vi "Write ModuleWidth.vi"(8 "error in (no error)":errorcluster, 10 "ModuleWidth":u8, 11 "Linear Barcode in":refnum<class "Linear Barcode.lvclass">) -> (0 "error out":errorcluster, 3 "Linear Barcode out":refnum<class "Linear Barcode.lvclass">)   [LabVIEW 2013, in "BarCodes.lvlib" / "Linear Barcode.lvclass"]
uses:
  Linear Barcode.lvclass
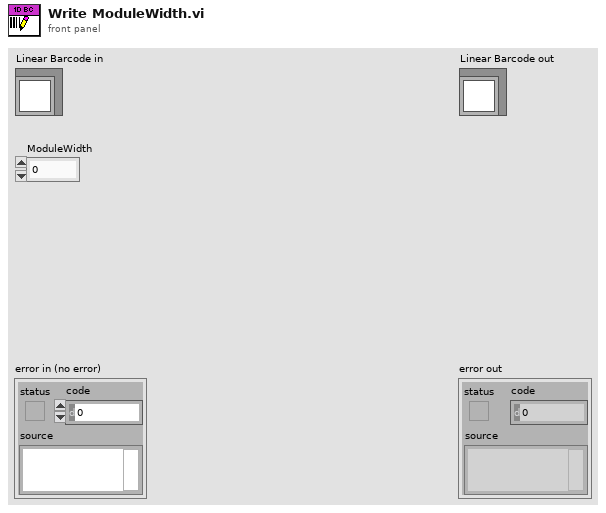
[diagram p1: front panel]
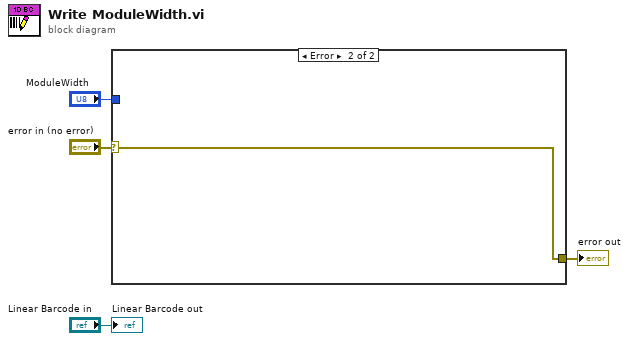
[diagram p0: block diagram]
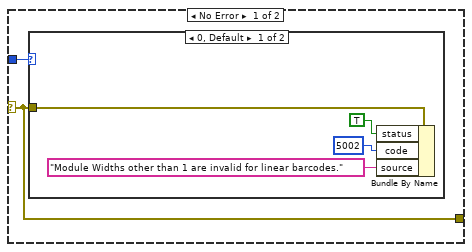
[diagram p2: hidden frame]
diagram:
  n1 = case shown="Error" "error in (no error)" {
    selector: "error in (no error)" -> [w5 w11]
    tunnel: "ModuleWidth" -> [w6 _]
    tunnel: [w5 w11] -> w2
    frame No Error {
      n2 = case shown="0, Default" w6 {
        tunnel: w5 -> [w10 _]
        frame 0, Default {
          n3 = Bundle By Name(cluster=w10, "status"=TRUE, "code"=5002, "source"="Module Widths other than 1 are invalid for linear barcodes.") -> ()  [unwired: 1 out]
        }
        frame 1 {
        }
      }
    }
    frame Error {
    }
  }
  "error out" <- w2
  "Linear Barcode out" <- "Linear Barcode in"
